vi "ChosseReceptorPass.vi"(6 "atacando ao contrário?":bool=TRUE, 8 "Impulso 2nd\nStriker Ativo":bool=TRUE, 10 "IA State Input":T2={"our_robots"=[], "enemy_robots"=[], "balls"=[], "geometry"={"line_width"=0, "field_length"=0, "field_width"=0, "boundary_width"=0, "referee_width"=0, "goal_width"=0, "goal_depth"=0, "goal_wall_width"=0, "center_circle_radius"=0, "defense_radius"=0, "defense_stretch"=0, "free_kick_from_defense_dist"=0, "penalty_spot_from_field_line_dist"=0, "penalty_line_from_spot_dist"=0}, "IA Judge"={"stage"="", "command"="", "our_goalie_id"=0.0, "enemy_goalie_id"=0.0, "command enum"=enum."Halt", "Time"=enum."Azul"}, "Received Timestamp"=timestamp(0 s since 1904-01-01), "Events"={"Touch"=FALSE, "Ball out"=FALSE, "id touch"=0.0, "Ball out of \nVision"=FALSE, "Ball inside \nGoalie area"=FALSE, "Robot not responding"=FALSE, "Robots responding status"=[1.0, 1.0, 1.0, 1.0, 1.0, 1.0], "Enemy Ball \nPossession"=FALSE, "Pass State"=FALSE, "id end of pass"=0.0, "Kick"=FALSE, "Id ini Possession"=0.0, "Ball Possesion"=FALSE, "Id Possesion"=0.0, "Direct Kick"=FALSE, "2nd Strk Ativo"=FALSE}}, 11 "AI Parameters":T1={"GotoKick"={"Dist do cone a frente"=150.0, "attacker farback"=1500.0, "Perto"=300.0, "min dist to kick"=150.0, "kick eps"=0.0, "Time to transition"=0.05}, "Attacker"={"CC chute"=0.09, "CC passe"=0.045, "Kick Force"=100.0, "ball-robot Kick"=200.0, "ball-robot Pass"=0.3, "drible\nAttk"=FALSE}, "Defender"={"D max"=1700.0, "Vel p/ robô av"=1000.0, "Kick Force"=100.0, "D atk-def"=0.0, "D farback"=0.0, "drible\ndef"=FALSE, "drible\ngoalie"=FALSE}, "Timeout"={"Field/v in x"=6.0, "Dist Robots"=300, "Dist up in y"=300}, "Pose Striker"={"dist"=200.0, "Numeric"=-4.0, "dist 2"=200.0, "drible\nstriker"=FALSE}, "Dist Stop"=300.0, "D ball out"=200, "D central gap "=150.0, "T pass"=0.0, "Force ++"=0.0, "range kick"=0.0, "Chute alto"=TRUE, "Marcador novo"=TRUE, "drible"=FALSE, "D drible"=300.0, "Versão Striker"=enum."3", "Defesa"=enum."ManMark", "Marcador"=enum."Marcar Segndo mais perigoso", "Receptor passe"=enum."2nd Striker", "Área"=enum."Quadrada"} {"D drible" format="%#_13g"; "D central gap" format="%#_13g"; "Dist Stop" format="%#_13g"; "Pose Striker"."Numeric" format="%#_13g"; "Defender"."Kick Force" format="%#_13g"; "Defender"."Vel p/ robô av" format="%#_13g"; "Attacker"."ball-robot Kick" format="%#_13g"; "Attacker"."Kick Force" format="%#_13g"; "Attacker"."CC passe" format="%#_13g"; "Attacker"."CC chute" format="%#_13g"; "GotoKick"."kick eps" format="%#_13g"; "GotoKick"."min dist to kick" format="%#_13g"; "GotoKick"."Perto" format="%#_13g"; "GotoKick"."attacker farback" format="%#_13g"; "GotoKick"."Dist do cone a frente" format="%#_13g"}) -> (3 "Receptor passe":enum16{"Auto", "2nd Striker", "Striker"}(ring)=enum."Striker")   [LabVIEW 2017]
uses:
  Core/AI Input.ctl
  Core/AI Robot.ctl
  Functions Enum.ctl
  AttackerStates.ctl
  Path Planning/RRT/PathDests.ctl
  Path Planning/RRT/PathDest.ctl
  Core/AI Ball.ctl
  Core/Field Size.ctl
  Core/AI Judge.ctl
  Command Enum.ctl
  Util/Events/Events.ctl
  AI Parameters.ctl
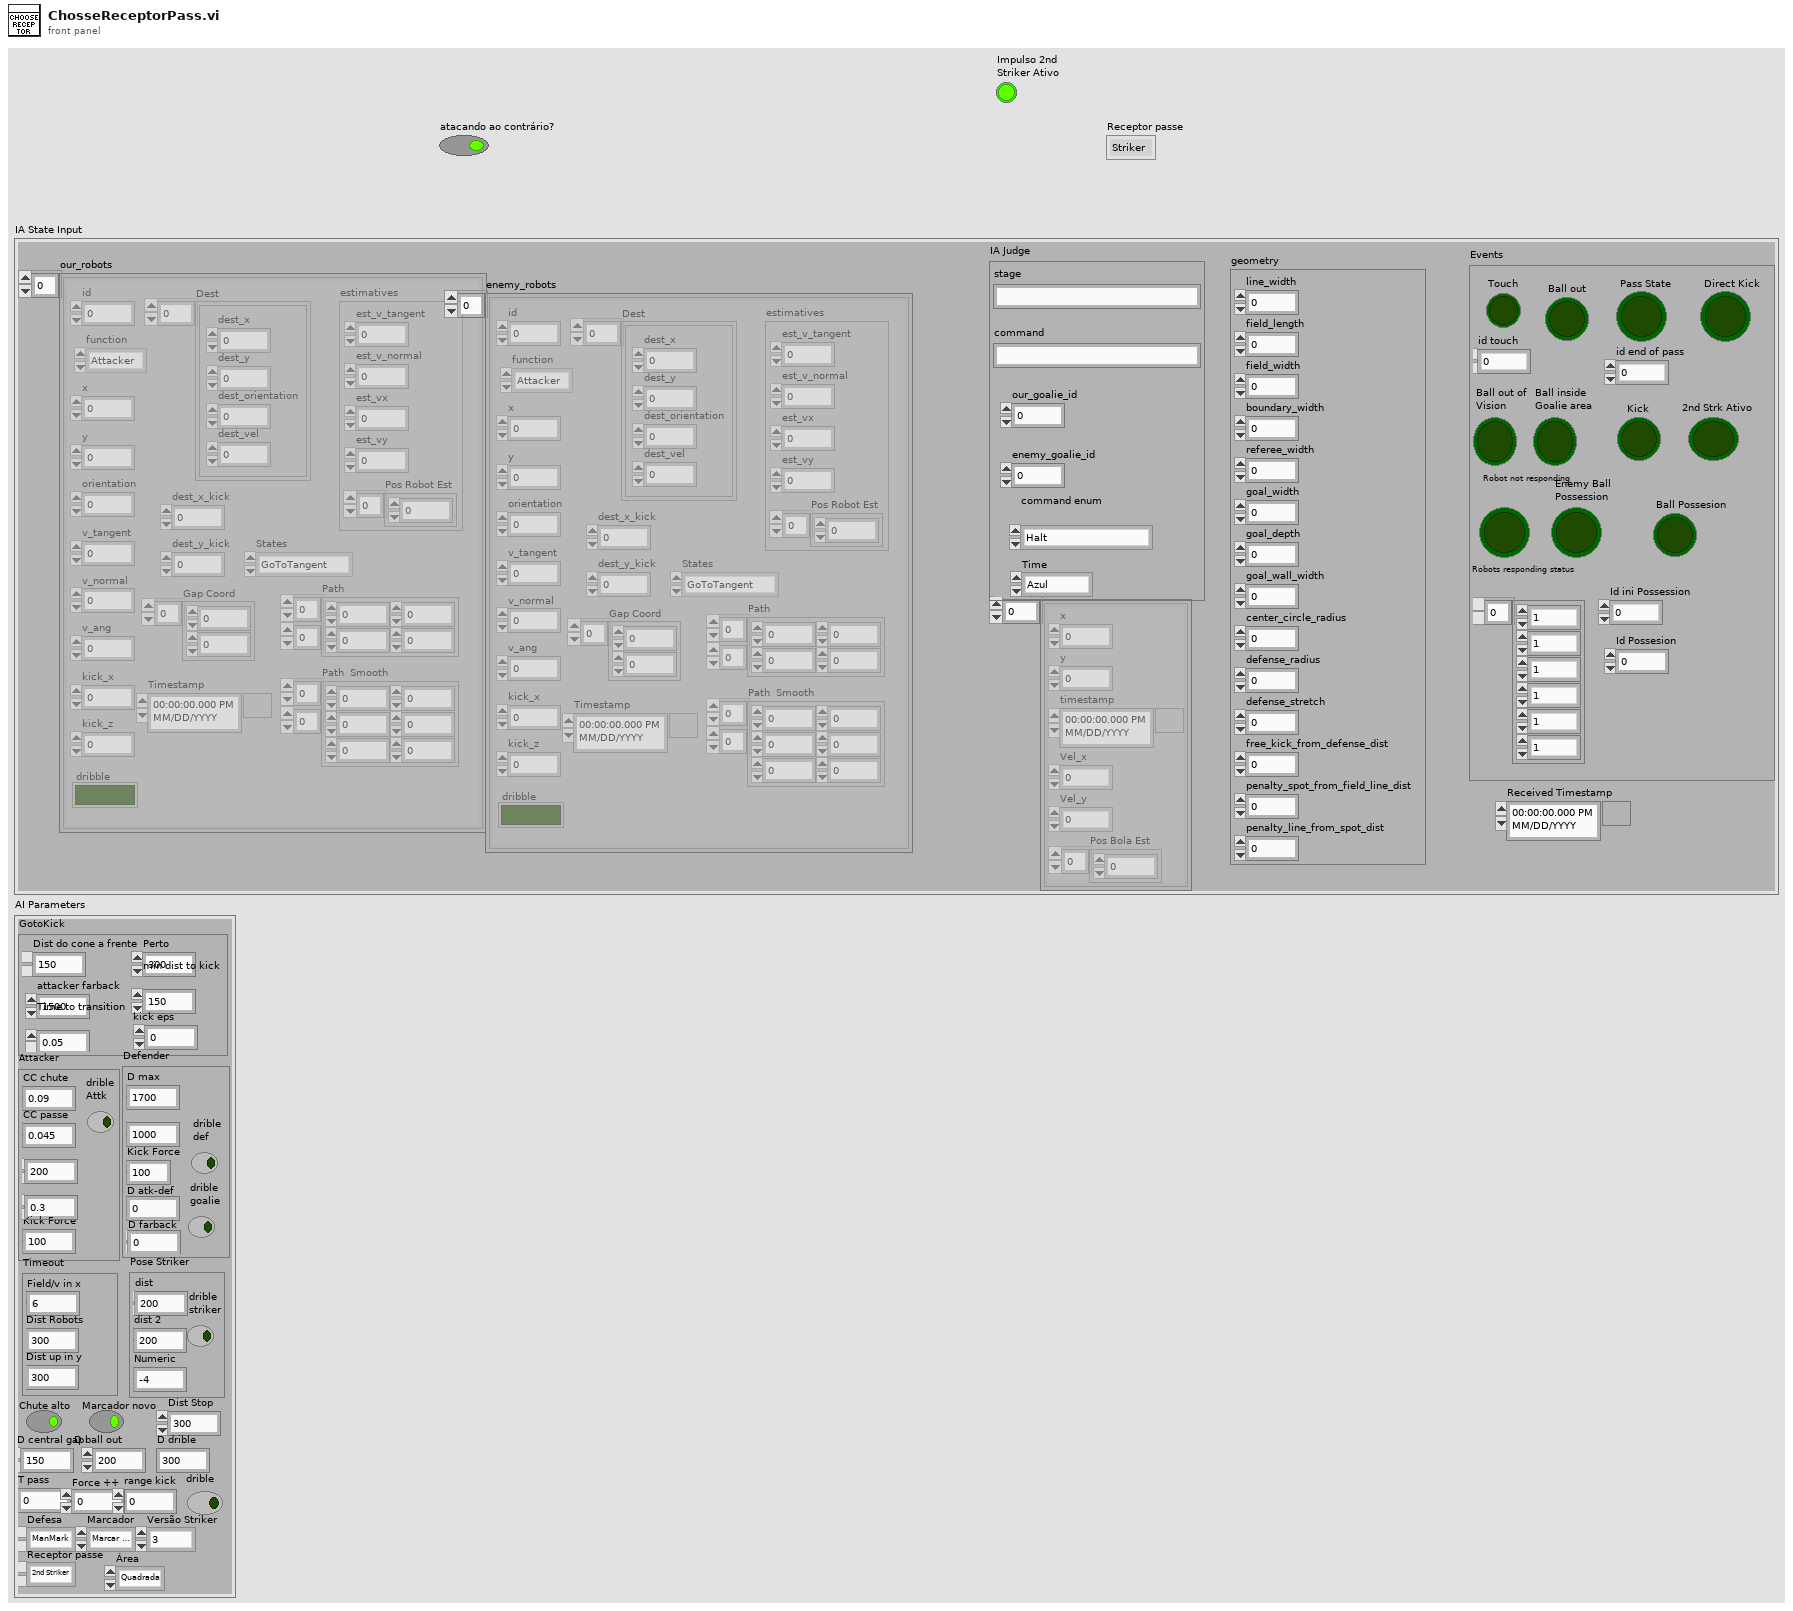
[diagram p1: front panel]
types:
  T1 = typedef "AI Parameters.ctl" = cluster{"GotoKick":cluster{"Dist do cone a frente":dbl, "attacker farback":dbl, "Perto":dbl, "min dist to kick":dbl, "kick eps":dbl, "Time to transition":dbl}, "Attacker":cluster{"CC chute":dbl, "CC passe":dbl, "Kick Force":dbl, "ball-robot Kick":dbl, "ball-robot Pass":dbl, "drible\nAttk":bool}, "Defender":cluster{"D max":dbl, "Vel p/ robô av":dbl, "Kick Force":dbl, "D atk-def":dbl, "D farback":dbl, "drible\ndef":bool, "drible\ngoalie":bool}, "Timeout":cluster{"Field/v in x":dbl, "Dist Robots":u32, "Dist up in y":u32}, "Pose Striker":cluster{"dist":dbl, "Numeric":dbl, "dist 2":dbl, "drible\nstriker":bool}, "Dist Stop":dbl, "D ball out":i32, "D central gap ":dbl, "T pass":dbl, "Force ++":dbl, "range kick":dbl, "Chute alto":bool, "Marcador novo":bool, "drible":bool, "D drible":dbl, "Versão Striker":enum16{"Auto", "3", "2", "1"}, "Defesa":enum16{"ManMark", "Barreira"}, "Marcador":enum16{"Marcar Segndo mais perigoso", "Marcar o mais perigoso"}, "Receptor passe":enum16{"Auto", "2nd Striker", "Striker"}, "Área":enum16{"Quadrada", "Circular"}}
  T2 = typedef "AI Input.ctl" = cluster{"our_robots":T3[], "enemy_robots":T3[], "balls":T8[], "geometry":T9, "IA Judge":T10, "Received Timestamp":timestamp, "Events":T12}
  T3 = typedef "AI Robot.ctl" = cluster{"id":u32, "function":T4, "x":dbl, "y":dbl, "orientation":dbl, "v_tangent":dbl, "v_normal":dbl, "v_ang":dbl, "kick_x":dbl, "kick_z":dbl, "dribble":bool, "Timestamp":timestamp, "estimatives":cluster{"est_v_tangent":dbl, "est_v_normal":dbl, "est_vx":dbl, "est_vy":dbl, "Pos Robot Est":dbl[]}, "dest_x_kick":dbl, "dest_y_kick":dbl, "Gap Coord":dbl[], "States":T5, "Path ":dbl[][], "Path  Smooth":dbl[][], "Dest":T6}
  T4 = typedef "Functions Enum.ctl" = enum16{"2nd Striker", "Attacker", "Goalie", "Defender", "Striker", "Goto 0", "Dummy", "Kicker", "ZigZag 0", "ZigZag 1", "ZigZag 2", "ZigZag 3", "ZigZag 4", "ZigZag 5", "ZigZag 6", "ZigZag 7", "ZigZag 8", ""}
  T5 = typedef "AttackerStates.ctl" = enum16{"Pass", "GoToTangent", "BallGetting", "GoToKick", ""}
  T6 = typedef "PathDests.ctl" = T7[]
  T7 = typedef "PathDest.ctl" = cluster{"dest_x":dbl, "dest_y":dbl, "dest_orientation":dbl, "dest_vel":dbl}
  T8 = typedef "AI Ball.ctl" = cluster{"x":dbl, "y":dbl, "timestamp":timestamp, "Vel_x":dbl, "Vel_y":dbl, "Pos Bola Est":dbl[]}
  T9 = typedef "Field Size.ctl" = cluster{"line_width":u32, "field_length":u32, "field_width":u32, "boundary_width":u32, "referee_width":u32, "goal_width":u32, "goal_depth":u32, "goal_wall_width":u32, "center_circle_radius":u32, "defense_radius":u32, "defense_stretch":u32, "free_kick_from_defense_dist":u32, "penalty_spot_from_field_line_dist":u32, "penalty_line_from_spot_dist":u32}
  T10 = typedef "AI Judge.ctl" = cluster{"stage":string, "command":string, "our_goalie_id":dbl, "enemy_goalie_id":dbl, "command enum":T11, "Time":enum16{"Azul", "Amarelo"}}
  T11 = typedef "Command Enum.ctl" = enum16{"Halt", "Stop", "Force Start", "PKA Normal Start", "Prepare Kickoff Ally", "PKE Normal Start", "Prepare Kickoff Enemy", "Prepare Penalty Ally", "PPA Normal Start", "Prepare Penalty Enemy", "PPE Normal Start", "Direct Free Enemy", "Direct Free Ally", "Indirect Free Enemy", "Indirect Free Ally", "Timeout Enemy", "Timeout Ally", "Goal Enemy", "Goal Ally", "Ball Placement Enemy", "Ball Placement Ally", "Normal Half Time", "Extra Time Break", "Extra Half Time", "None", "Post Game"}
  T12 = typedef "Events.ctl" = cluster{"Touch":bool, "Ball out":bool, "id touch":dbl, "Ball out of \nVision":bool, "Ball inside \nGoalie area":bool, "Robot not responding":bool, "Robots responding status":dbl[], "Enemy Ball \nPossession":bool, "Pass State":bool, "id end of pass":dbl, "Kick":bool, "Id ini Possession":dbl, "Ball Possesion":bool, "Id Possesion":dbl, "Direct Kick":bool, "2nd Strk Ativo":bool}
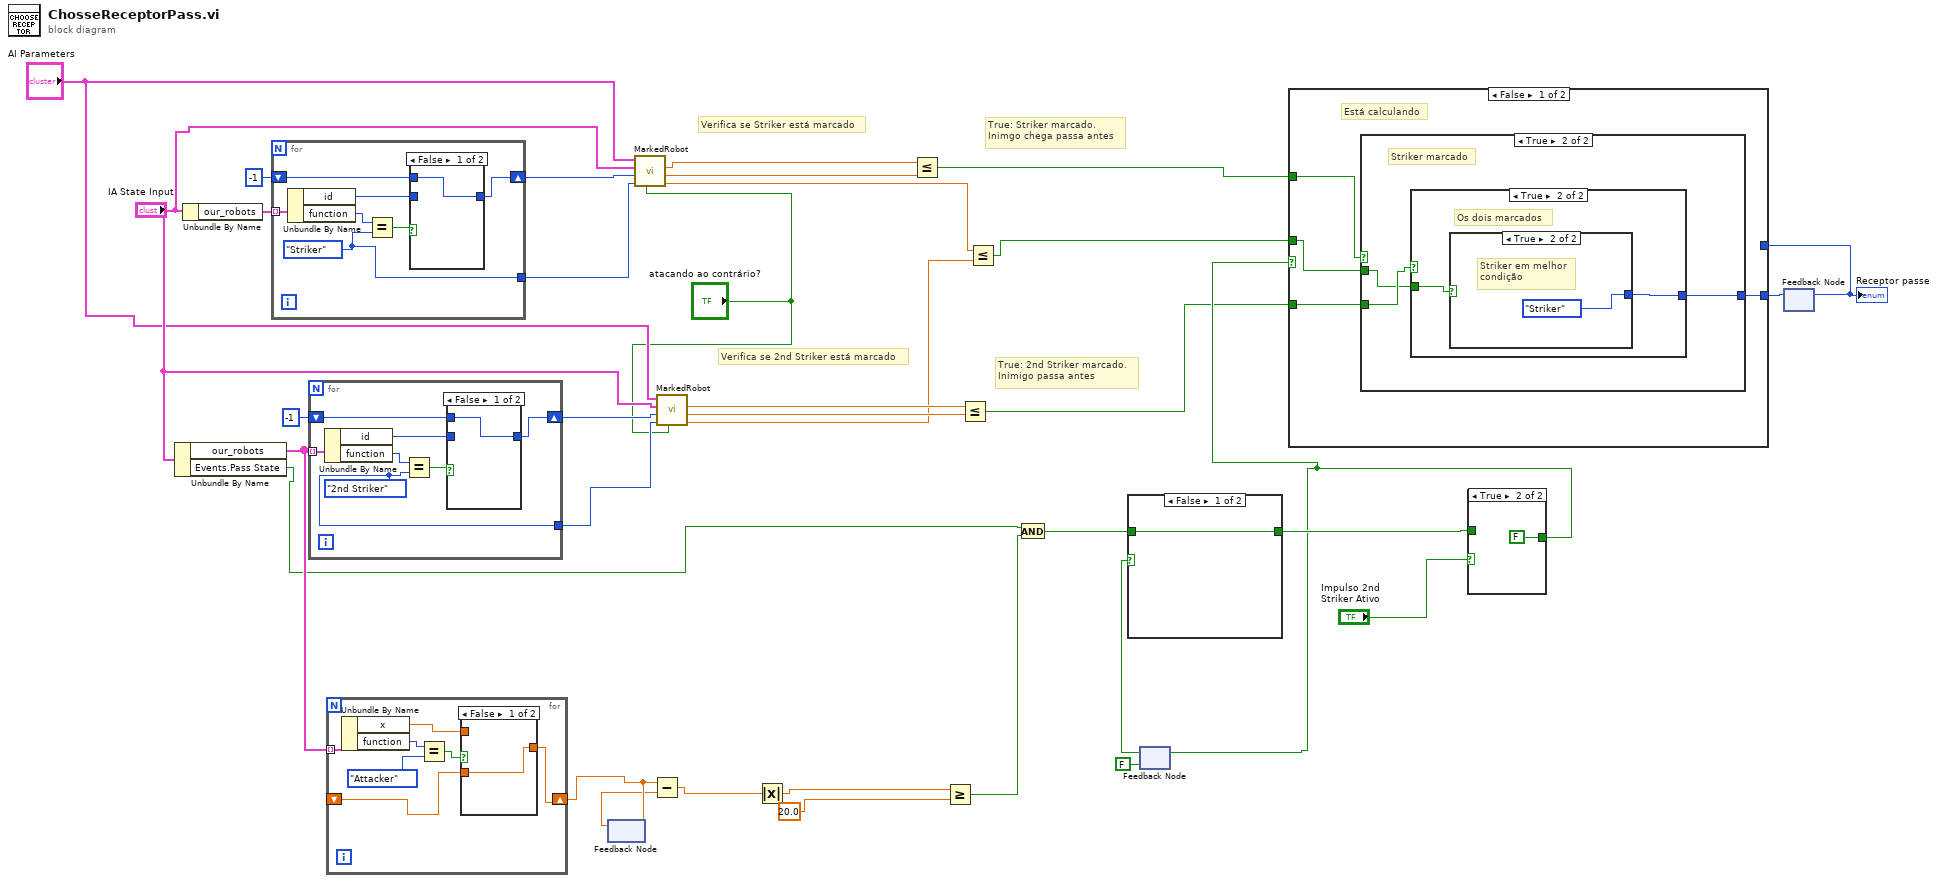
[diagram p0: block diagram]
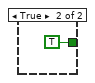
[diagram p3: hidden frame]
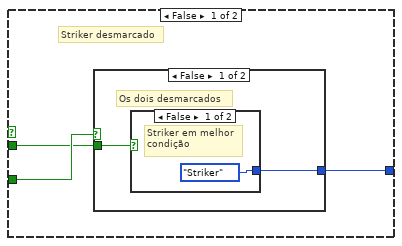
[diagram p5: hidden frame]
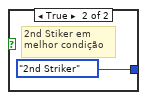
[diagram p6: hidden frame]
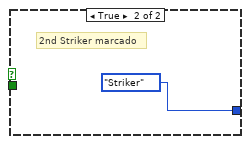
[diagram p7: hidden frame]
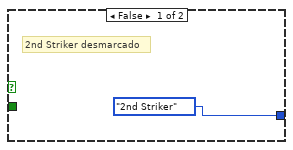
[diagram p8: hidden frame]
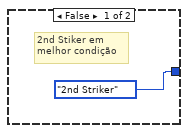
[diagram p9: hidden frame]
diagram:
  # "True: 2nd Striker marcado.\nInimigo passa antes"
  # "True: Striker marcado.\nInimgo chega passa antes"
  # "Verifica se 2nd Striker está marcado"
  # "Verifica se Striker está marcado"
  n1 = Unbundle By Name("IA State Input") -> ("our_robots"=w26:T3[], "Events.Pass State"=w17:bool)
  n2 = Unbundle By Name("IA State Input") -> ("our_robots"=w35:T3[])
  n3 = for {
    tunnel: w35 -> [w42] mode=indexing
    shift-right: [w39] -> w33
    shift-left: -1 ("id") -> [w37]
    tunnel: [w36] -> w13
    w36 = Functions_Enum."Striker" ("y")
    n4 = Unbundle By Name(w42) -> ("id"=w38:u32, "function"=w41:T4)
    n5 = Equal?(x=w41, y=w36) -> (x = y?=w40:bool)
    n6 = case shown="False" w40 {
      tunnel: [w43 w44] -> w39
      tunnel: w38 -> [_ w44]
      tunnel: w37 -> [w43 _]
      frame False {
      }
      frame True {
      }
    }
  }
  n7 = for {
    tunnel: w26 -> [w51] mode=indexing
    shift-right: [w48] -> w31
    shift-left: -1 ("id") -> [w46]
    tunnel: [w45] -> w14
    w45 = Functions_Enum."2nd Striker" ("y")
    n8 = Unbundle By Name(w51) -> ("id"=w47:u32, "function"=w50:T4)
    n9 = Equal?(x=w50, y=w45) -> (x = y?=w49:bool)
    n10 = case shown="False" w49 {
      tunnel: [w52 w53] -> w48
      tunnel: w47 -> [_ w53]
      tunnel: w46 -> [w52 _]
      frame False {
      }
      frame True {
      }
    }
  }
  n11 = for {
    tunnel: w26 -> [w60] mode=indexing
    shift-right: [w56] -> w25
    shift-left: _ -> [w54]
    n12 = Unbundle By Name(w60) -> ("x"=w55:dbl, "function"=w59:T4)
    n13 = Equal?(x=w59, y=Functions_Enum."Attacker") -> (x = y?=w57:bool)
    n14 = case shown="False" w57 {
      tunnel: [w61 w62] -> w56
      tunnel: w55 -> [_ w62]
      tunnel: w54 -> [w61 _]
      frame False {
      }
      frame True {
      }
    }
  }
  n15 = feedback-in #1(w25) -> ()
  n16 = feedback #1() -> (w24:dbl)  [unwired: 1 in]
  n17 = call "MarkedRobot.vi"("atacando ao contrário?"="atacando ao contrário?", "Função"=w13, "id"=w33, "IA State Input"="IA State Input", "AI Parameters"="AI Parameters") -> ("Dif. tempo inimigo\ntempo bola"=w3:dbl, "Tempo p/ bola\npassar pelo ponto"=w8:dbl, "Tempo p/ inimigo\nchegar à reta"=w9:dbl)  [unwired: 3 in, 1 out]
  n18 = Subtract(x=w25, y=w24) -> (x-y=w23:dbl)
  n19 = call "MarkedRobot.vi"("atacando ao contrário?"="atacando ao contrário?", "Função"=w14, "id"=w31, "IA State Input"="IA State Input", "AI Parameters"="AI Parameters") -> ("Dif. tempo inimigo\ntempo bola"=w2:dbl, "Tempo p/ bola\npassar pelo ponto"=w5:dbl, "Tempo p/ inimigo\nchegar à reta"=w6:dbl)  [unwired: 3 in, 1 out]
  n20 = Absolute Value(x=w23) -> (abs(x)=w22:dbl)
  n21 = Less Or Equal?(x=w9, y=w8) -> (x <= y?=w7:bool)
  n22 = Greater Or Equal?(x=w22, y=20.0) -> (x >= y?=w20:bool)
  n23 = Less Or Equal?(x=w6, y=w5) -> (x <= y?=w4:bool)
  n24 = Less Or Equal?(x=w3, y=w2) -> (x <= y?=w1:bool)
  n25 = And(x=w17, y=w20) -> (x .and. y?=w18:bool)
  n26 = feedback #2(FALSE) -> (w11:bool)
  n27 = case shown="False" w11 {
    tunnel: [w63 TRUE] -> w16
    tunnel: w18 -> [w63 _]
    frame False {
    }
    frame True {
    }
  }
  n28 = case shown="True" "Impulso 2nd\nStriker Ativo" {
    tunnel: [w65 FALSE] -> w15
    tunnel: w16 -> [w65 _]
    frame False {
    }
    frame True {
    }
  }
  n29 = feedback-in #2(w15) -> ()
  n30 = feedback #3() -> (w27:enum16{"Auto", "2nd Striker", "Striker"})  [unwired: 1 in]
  "Receptor passe" <- w27
  n31 = case shown="False" w15 {
    tunnel: [w70 w87] -> w28
    tunnel: w27 -> [_ w87]
    tunnel: w7 -> [w69 _]
    tunnel: w4 -> [w68 _]
    tunnel: w1 -> [w67 _]
    frame False {
      # "Está calculando"
      n32 = case shown="True" w69 {
        tunnel: [w73 w81] -> w70
        tunnel: w68 -> [w72 w80]
        tunnel: w67 -> [w71 w79]
        frame False {
          # "Striker desmarcado"
          n33 = case shown="False" w72 {
            tunnel: [w74 enum16{"Auto", "2nd Striker", "Striker"}."Striker" ("Receptor passe")] -> w73
            tunnel: w71 -> [w75 _]
            frame False {
              # "Os dois desmarcados"
              n34 = case shown="False" w75 {
                tunnel: [enum16{"Auto", "2nd Striker", "Striker"}."Striker" ("Receptor passe") enum16{"Auto", "2nd Striker", "Striker"}."2nd Striker" ("Receptor passe")] -> w74
                frame False {
                  # "Striker em melhor\ncondição"
                }
                frame True {
                  # "2nd Stiker em\nmelhor condição"
                }
              }
            }
            frame True {
              # "2nd Striker marcado"
            }
          }
        }
        frame True {
          # "Striker marcado"
          n35 = case shown="True" w80 {
            tunnel: [enum16{"Auto", "2nd Striker", "Striker"}."2nd Striker" ("Receptor passe") w83] -> w81
            tunnel: w79 -> [_ w84]
            frame False {
              # "2nd Striker desmarcado"
            }
            frame True {
              # "Os dois marcados"
              n36 = case shown="True" w84 {
                tunnel: [enum16{"Auto", "2nd Striker", "Striker"}."2nd Striker" ("Receptor passe") enum16{"Auto", "2nd Striker", "Striker"}."Striker" ("Receptor passe")] -> w83
                frame False {
                  # "2nd Stiker em\nmelhor condição"
                }
                frame True {
                  # "Striker em melhor\ncondição"
                }
              }
            }
          }
        }
      }
    }
    frame True {
      # "Já parou de calcular"
    }
  }
  n37 = feedback-in #3(w28) -> ()
